vi "Actor Core.vi"(8 "error in":errorcluster, 11 "Instrument.lvclass":refnum<class "Instrument.lvclass">) -> (0 "error out":errorcluster, 3 "Actor":refnum<class "Actor.lvclass">)   [LabVIEW 2015, in "Item Actor.lvlib" / "Instrument.lvclass"]
uses:
  Instrument.lvclass
  <vilib>/ActorFramework/Actor/Actor.lvclass
  Instrument.lvclass/Instrument.ctl
  Read Description.vi
  Read Owner.vi
  Read Version.vi
  Read Preview2.vi
  Generic Item/Generic Item.lvclass
panel:
  out "Name":string
  out "Version:":string
  out "Description:":string
  out "Dev/Company:":string
  out "Preview":picture
  in  "Run when opened:":bool
  out "Instrument Type:":string
  in  "Launch":bool
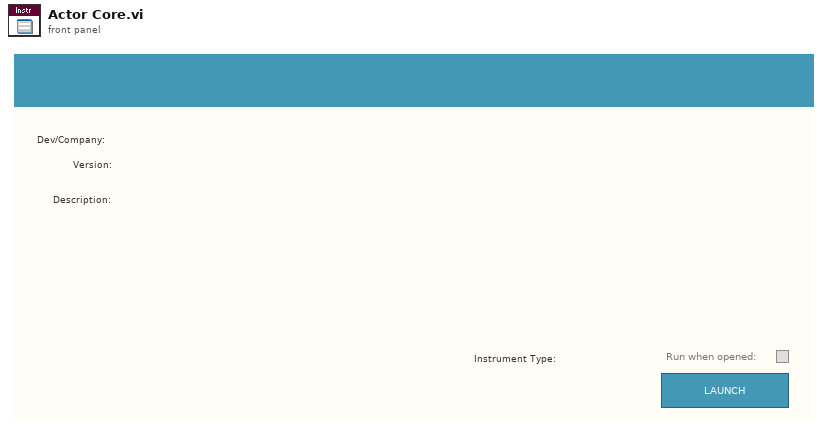
[diagram p1: front panel]
types:
  T1 = enum8{"Enabled", "Disabled", "Disabled and Grayed Out"}
  T2 = typedef "imagedata.ctl" = cluster{"image type":i32, "image depth":i32, "image":u8[], "mask":u8[], "colors":u32[], "Rectangle":cluster{"left":i16, "top":i16, "right":i16, "bottom":i16}}
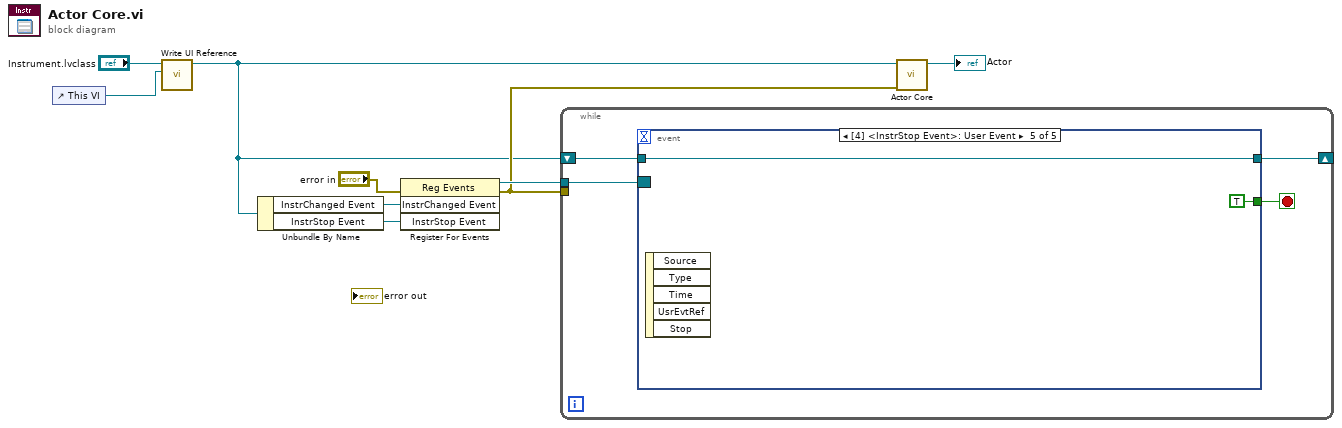
[diagram p0: block diagram]
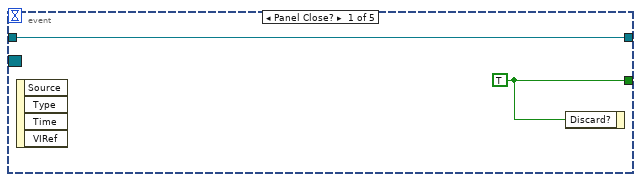
[diagram p2: hidden frame]
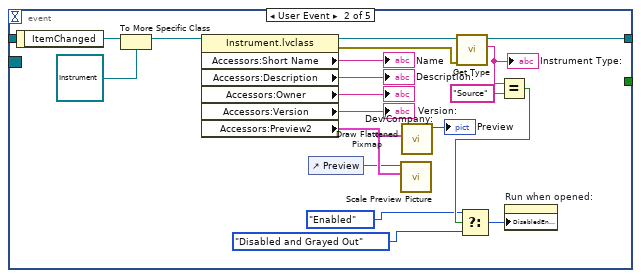
[diagram p3: hidden frame]
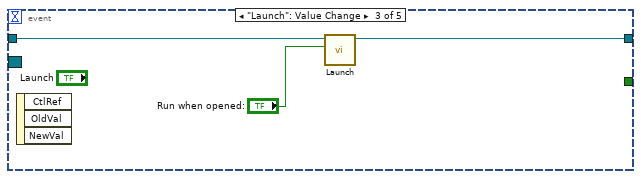
[diagram p4: hidden frame]
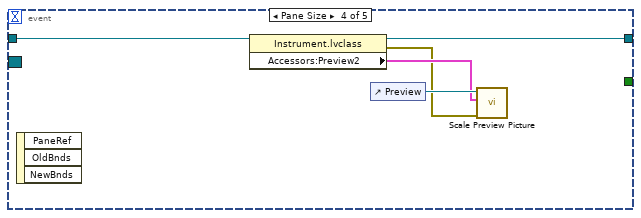
[diagram p5: hidden frame]
diagram:
  n1 = control-ref of="This VI"() -> (w1:refnum<vi>)
  n2 = call "Write UI Reference.vi"("Item Panel"=w1, "Generic Item in"="Instrument.lvclass") -> ("Generic Item out"=w2:refnum<class "Instrument.lvclass">)  [unwired: 8 in, 1 out]
  n3 = Unbundle By Name(w2) -> ("InstrChanged Event"=w5:refnum<user-event>, "InstrStop Event"=w4:refnum<user-event>)
  n4 = register-events(error in="error in", w5, w4) -> (reference out=w9:refnum<event-registration>, error out=w6:errorcluster)  [unwired: 1 in]
  n5 = while {
    tunnel: w9 -> [w13]
    shift-right: [w11] -> _
    shift-left: w2 -> [w10]
    tunnel: w6 -> [_]
    stop <- w12 stop-if-true
    n6 = event shown="[4] <InstrStop Event>: User Event" {
      selector: w13 -> [_ _ _ _ _]
      dyn-events: _ -> [_ _ _ _ _]
      timeout: _ -> [_ _ _ _ _]
      tunnel: [w15 _ _ _ TRUE ("Discard?")] -> w12
      tunnel: [w14 w28 w36 w38 w44] -> w11
      tunnel: w10 -> [w14 _ w37 w41 w44]
      event Panel Close? {
        w15 = TRUE ("Discard?")
        n7 = event-data() -> ()  [unwired: 1 in, 4 out]
        n8 = event-data("Discard?"=w15) -> ()  [unwired: 1 in, 1 out]
      }
      event User Event {
        n9 = event-data() -> ("ItemChanged"=w20:refnum<class "Generic Item.lvclass">)  [unwired: 1 in]
        n10 = To More Specific Class(target class=refnum<class "Instrument.lvclass"> refnum ("Instrument.lvclass"), reference=w20) -> (specific class reference=w18:refnum<class "Instrument.lvclass">)  [unwired: 1 in, 1 out]
        n11 = property class="Instrument.lvclass"(reference=w18) -> (reference out=w17:refnum<class "Instrument.lvclass">, error out=w16:errorcluster, "Accessors:Short Name"=→"Name":string, "Accessors:Description"=→"Description:":string, "Accessors:Owner"=→"Dev/Company:":string, "Accessors:Version"=→"Version:":string, "Accessors:Preview2"=w30:T2)  [unwired: 1 in]
        n12 = control-ref of="Preview"() -> (w29:refnum<vi>)
        n13 = call "Scale Preview Picture.vi"("Accessors:Preview2"=w30, "Picture in"=w29) -> ()  [unwired: 9 in, 1 out]
        n14 = call <vilib>:"Draw Flattened Pixmap.vi"("image data"=w30) -> ("new picture"=→"Preview":picture)  [unwired: 8 in]
        n15 = call-dynamic "Get Type.vi"("error in (no error)"=w16, "Instrument in"=w17) -> ("Type"=w27:string, "Instrument out"=w28:refnum<class "Instrument.lvclass">)  [unwired: 7 in, 1 out]
        "Instrument Type:" <- w27
        n16 = Equal?(x=w27, y="Source") -> (x = y?=w25:bool)
        n17 = Select(t=T1."Enabled" ("Disabled"), s=w25, f=T1."Disabled and Grayed Out" ("Disabled")) -> (s? t:f=w22:T1)
        n18 = property on="Run when opened:" class="Bool (strict)"("DisabledEnum"=w22) -> ()  [unwired: 2 in, 2 out]
      }
      event "Launch": Value Change {
        n19 = event-data() -> ()  [unwired: 1 in, 3 out]
        n20 = call-dynamic "Launch.vi"("Run"="Run when opened:", "Instrument in"=w37) -> ("Instrument out"=w36:refnum<class "Instrument.lvclass">)  [unwired: 8 in, 1 out]
      }
      event Pane Size {
        n21 = event-data() -> ()  [unwired: 1 in, 3 out]
        n22 = property class="Instrument.lvclass"(reference=w41) -> (reference out=w38:refnum<class "Instrument.lvclass">, error out=w39:errorcluster, "Accessors:Preview2"=w40:T2)  [unwired: 1 in]
        n23 = control-ref of="Preview"() -> (w42:refnum<vi>)
        n24 = call "Scale Preview Picture.vi"("error in (no error)"=w39, "Accessors:Preview2"=w40, "Picture in"=w42) -> ()  [unwired: 8 in, 1 out]
      }
      event User Event {
        n25 = event-data() -> ()  [unwired: 1 in, 5 out]
      }
    }
  }
  n26 = call-parent "Actor Core.vi"("error in"=w6, "Generic Item in"=w2) -> ("Actor out"=→"Actor":refnum<class "Actor.lvclass">)  [unwired: 8 in, 1 out]
